vi "PopulatePortsAndSpeedsGain.vi"(9 "Ports and Speeds":refnum<vi>, 10 "Gain":refnum<vi>, 11 ".NET Refnum in":refnum<k24>) -> ()   [LabVIEW 2018]
uses:
  D:/SVN/PM/sdk/AppSamples/LabVIEWSamples/trunk/Release/2018/Dependencies/PVCamNET.dll
  Dependencies/PVCamNET.dll
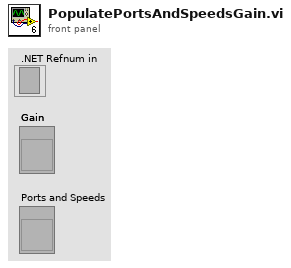
[diagram p1: front panel]
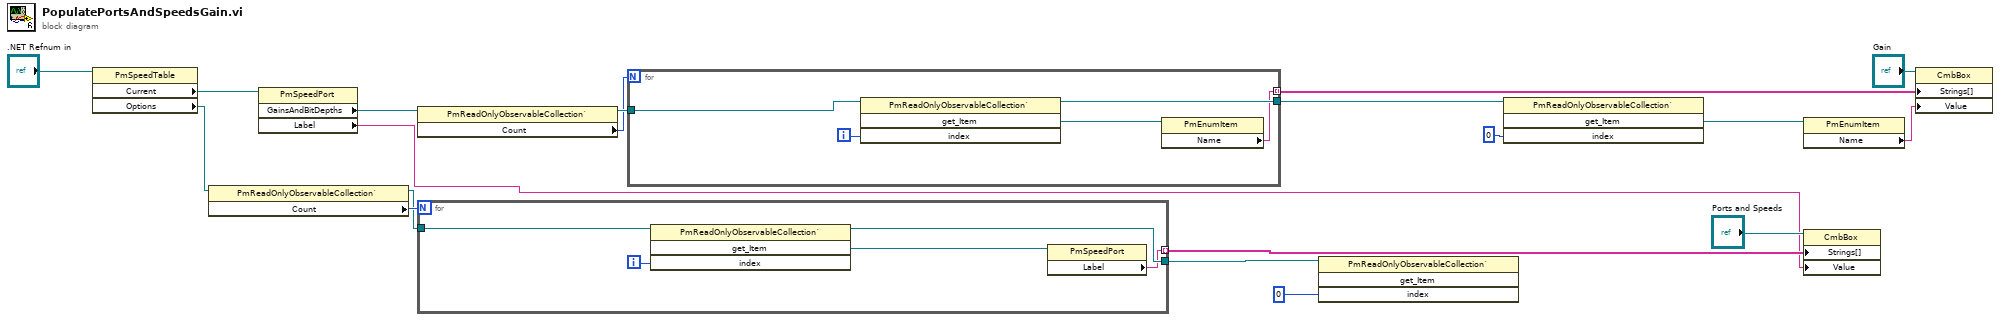
[diagram p0: block diagram]
diagram:
  n1 = property class="PmSpeedTable"(reference=".NET Refnum in") -> ("Current"=w3:refnum<k24>, "Options"=w12:refnum<k24>)  [unwired: 1 in, 2 out]
  n2 = property class="PmReadOnlyObservableCollection`"(reference=w12) -> (reference out=w13:refnum<k24>, "Count"=w14:i32)  [unwired: 1 in, 1 out]
  n3 = property class="PmSpeedPort"(reference=w3) -> ("GainsAndBitDepths"=w4:refnum<k24>, "Label"=w1:string)  [unwired: 1 in, 2 out]
  n4 = property class="PmReadOnlyObservableCollection`"(reference=w4) -> (reference out=w6:refnum<k24>, "Count"=w5:i32)  [unwired: 1 in, 1 out]
  n5 = for {
    N: w14 -> [_]
    tunnel: w13 -> [w24]
    tunnel: [w22] -> w18
    tunnel: [w20] -> w16 mode=indexing
    i -> [w23]
    n6 = invoke class="PmReadOnlyObservableCollection`" method="get_Item"(reference=w24, "index"=w23) -> (reference out=w22:refnum<k24>, "get_Item"=w21:refnum<k24>)  [unwired: 2 in, 2 out]
    n7 = property class="PmSpeedPort"(reference=w21) -> ("Label"=w20:string)  [unwired: 1 in, 2 out]
  }
  n8 = for {
    N: w5 -> [_]
    tunnel: w6 -> [w29]
    tunnel: [w26] -> w9
    tunnel: [w25] -> w11 mode=indexing
    i -> [w28]
    n9 = invoke class="PmReadOnlyObservableCollection`" method="get_Item"(reference=w29, "index"=w28) -> (reference out=w26:refnum<k24>, "get_Item"=w27:refnum<k24>)  [unwired: 2 in, 2 out]
    n10 = property class="PmEnumItem"(reference=w27) -> ("Name"=w25:string)  [unwired: 1 in, 2 out]
  }
  n11 = invoke class="PmReadOnlyObservableCollection`" method="get_Item"(reference=w18, "index"=0) -> ()  [unwired: 2 in, 4 out]
  n12 = invoke class="PmReadOnlyObservableCollection`" method="get_Item"(reference=w9, "index"=0) -> ("get_Item"=w8:refnum<k24>)  [unwired: 2 in, 3 out]
  n13 = property class="PmEnumItem"(reference=w8) -> ("Name"=w19:string)  [unwired: 1 in, 2 out]
  n14 = property class="CmbBox"(reference="Ports and Speeds", "Strings[]"=w16, "Value"=w1) -> ()  [unwired: 1 in, 2 out]
  n15 = property class="CmbBox"(reference="Gain", "Strings[]"=w11, "Value"=w19) -> ()  [unwired: 1 in, 2 out]
